vi "19052 Get_FALL_time.vi"(7 "Mode":T1, 8 "error in (no error)":errorcluster, 9 "Step":u16=1 min=1 max=99 step=1, 11 "VISA resource in":refnum<visa-resource-name>) -> (0 "error out":errorcluster, 1 "FALL time":dbl format="%.1p", 3 "VISA resource out":refnum<visa-resource-name>)   [LabVIEW 2015]
uses:
  Type Definitions/ac_dc_ir_control.ctl
panel:
  out "output command":string
  # "Get FALL time"
  # "[s]"
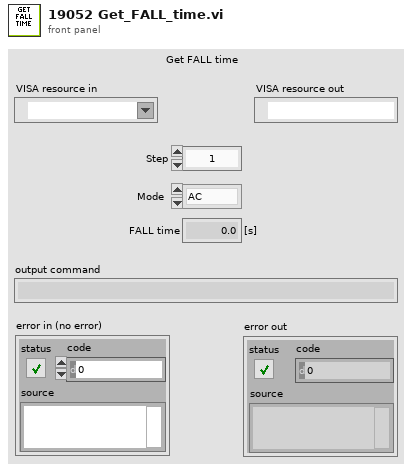
[diagram p1: front panel]
types:
  T1 = typedef "ac_dc_ir_control.ctl" = enum16{"AC", "DC", "IR"}
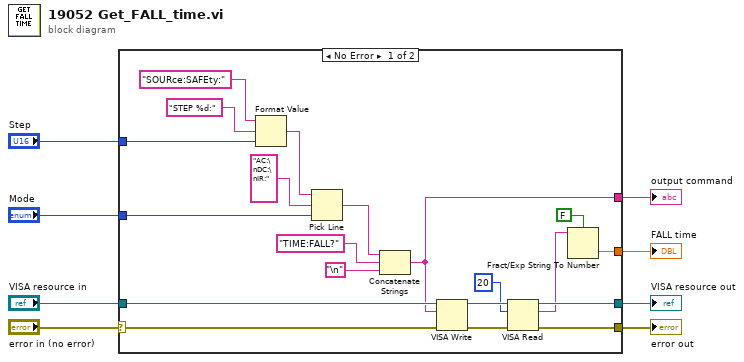
[diagram p0: block diagram]
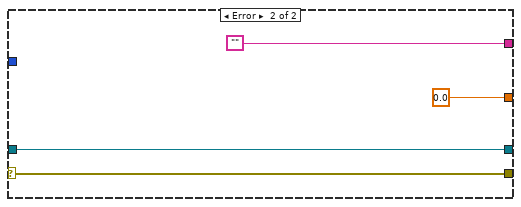
[diagram p2: hidden frame]
diagram:
  n1 = case shown="No Error" "error in (no error)" {
    selector: "error in (no error)" -> [w12 w30]
    tunnel: [w28 w30] -> w8
    tunnel: "VISA resource in" -> [w27 w32]
    tunnel: "Step" -> [w26 _]
    tunnel: [w18 ""] -> w6
    tunnel: [w14 w32] -> w5
    tunnel: "Mode" -> [w13 _]
    tunnel: [w11 0.0] -> w1
    frame No Error {
      n2 = Format Value(string ("")="SOURce:SAFEty:", format string="STEP %d:", value (0)=w26) -> (output string=w23:string)
      n3 = Pick Line(string ("")=w23, multi-line string="AC:\nDC:\nIR:", line index=w13) -> (output string=w20:string)
      n4 = Concatenate Strings(w20, "TIME:FALL?", "\n") -> (w18:string)
      n5 = VISA Write(VISA resource name=w27, write buffer=w18, error in (no error)=w12) -> (VISA resource name out=w16:refnum<visa-resource-name>, error out=w17:errorcluster)  [unwired: 1 out]
      n6 = VISA Read(VISA resource name=w16, byte count=u32 20, error in (no error)=w17) -> (VISA resource name out=w14:refnum<visa-resource-name>, read buffer=w10:string, error out=w28:errorcluster)  [unwired: 1 out]
      n7 = Fract/Exp String To Number(use system decimal point (T)=FALSE, string=w10) -> (number=w11:dbl)  [unwired: 2 in, 1 out]
    }
    frame Error {
    }
  }
  "error out" <- w8
  "VISA resource out" <- w5
  "output command" <- w6
  "FALL time" <- w1
